vi "createFromXMLNative.vi"(8 "error in (no error)":errorcluster, 10 "scriptEventXML":refnum<k20>) -> (0 "error out":errorcluster, 3 "ScriptEvent out":refnum<class "ScriptEvent.lvclass">)   [LabVIEW 2011, in "Tools.lvlib" / "Scripting.lvlib" / "ScriptEvent.lvclass"]
uses:
  ScriptEvent.lvclass
  <vilib>/xml/Close Reference(Node).vi
  <vilib>/xml/NI_XML.lvlib
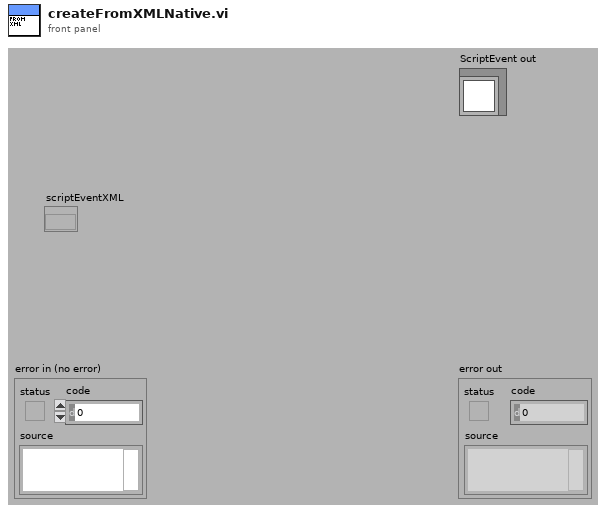
[diagram p1: front panel]
types:
  T1 = enum16{"changeValue", "pulse", "clock", "rampUp", "rampDown", "singleTone", "singleToneRamp", "playFile"}
  T2 = enum16{"changeValue", "pulse", "clock", "rampUp", "rampDown", "singleTone", "singleToneRamp", "playFile", "rf"}
  T3 = enum16{"changeValue", "pulse", "clock", "rampUp", "rampDown", "singleTone", "singleToneRamp", "playFile", "rf", "rfRamp"}
  T4 = enum16{"changeValue", "pulse", "clock", "rampUp", "rampDown", "singleTone", "singleToneRamp", "playFile", "rf", "rfRamp", "delay"}
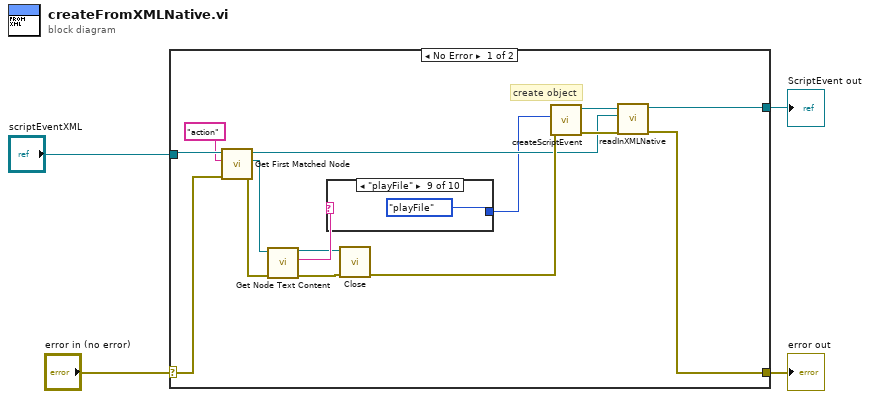
[diagram p0: block diagram]
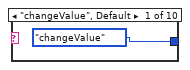
[diagram p2: hidden frame]
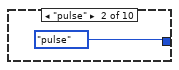
[diagram p3: hidden frame]
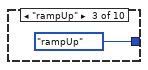
[diagram p4: hidden frame]
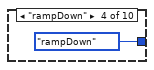
[diagram p5: hidden frame]
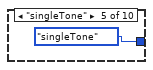
[diagram p6: hidden frame]
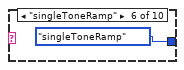
[diagram p7: hidden frame]
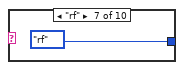
[diagram p8: hidden frame]
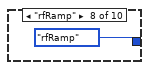
[diagram p9: hidden frame]
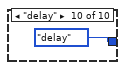
[diagram p10: hidden frame]
diagram:
  n1 = case shown="No Error" "error in (no error)" {
    selector: "error in (no error)" -> [w12 w30]
    tunnel: [w11 w30] -> w3
    tunnel: "scriptEventXML" -> [w19 _]
    tunnel: [w13 _] -> w1
    frame No Error {
      # "create object"
      n2 = call <vilib>:"Get First Matched Node.vi"("error in (no error)"=w12, "XPath expression"="action", "node in"=w19) -> ("error out"=w17:errorcluster, "node result"=w16:refnum<k20>, "node out"=w6:refnum<k20>)  [unwired: 6 in]
      n3 = call <vilib>:"Get Node Text Content.vi"("error in (no error)"=w17, "node in"=w16) -> ("error out"=w9:errorcluster, "node text"=w15:string, "node out"=w10:refnum<k20>)  [unwired: 7 in]
      n4 = case shown="\"playFile\"" w15 {
        tunnel: [T1."changeValue" ("action") T1."pulse" ("action") T1."rampUp" ("action") T1."rampDown" ("action") T1."singleTone" ("action") T1."singleToneRamp" ("action") T2."rf" ("action") T3."rfRamp" ("action") T3."playFile" ("action") T4."delay" ("action")] -> w5
        frame "changeValue", Default {
        }
        frame "pulse" {
        }
        frame "rampUp" {
        }
        frame "rampDown" {
        }
        frame "singleTone" {
        }
        frame "singleToneRamp" {
        }
        frame "rf" {
        }
        frame "rfRamp" {
        }
        frame "playFile" {
        }
        frame "delay" {
        }
      }
      n5 = call-poly <vilib>:"Close.vi"("error in (no error)"=w9, "node"=w10) -> ("error out"=w8:errorcluster)  [unwired: 7 in]
      n6 = call "createScriptEvent.vi"("error in (no error)"=w8, "action"=w5) -> ("error out"=w7:errorcluster, "ScriptEvent out"=w14:refnum<class "ScriptEvent.lvclass">)  [unwired: 8 in]
      n7 = call-dynamic "readInXMLNative.vi"("error in (no error)"=w7, "scriptEventXML"=w6, "ScriptEvent in"=w14) -> ("error out"=w11:errorcluster, "ScriptEvent out"=w13:refnum<class "ScriptEvent.lvclass">)  [unwired: 7 in]
    }
    frame Error {
    }
  }
  "error out" <- w3
  "ScriptEvent out" <- w1
